vi "长度判断.vi"(6 "输入元素 2":string, 8 "error in (no error)":errorcluster caption="错误输入（无错误）", 9 "压力打印代码据库":string[][](table)=[["C.0A.00D", "C.04.001", "C.0B.31B", ""], ["C.0A.01D", "C.04.002", "C.0B.32B", ""], ["C.0A.02D", "C.04.003", "C.0B.33B", ""], ["C.0A.03D", "C.04.004", "C.0B.34B", ""], ["C.0A.04D", "C.04.005", "C.0B.35B", ""], ["C.0A.05D", "C.04.006", "C.0B.36B", ""], ["C.0A.06D", "C.04.007", "C.0B.37B", ""], ["C.0A.07D", "C.04.008", "C.0B.38B", ""], ["C.0A.08D", "C.04.009", "C.0B.39B", ""], ["C.0A.09D", "C.04.010", "C.0B.3AB", ""], ["C.0A.0AD", "C.04.011", "C.0B.3BB", ""], ["C.0A.0BD", "C.04.012", "C.0B.3CB", ""], ["C.0A.0CD", "C.04.013", "C.0B.1MB", ""], ["C.0A.0DD", "C.04.014", "C.0B.1NB", ""], ["C.0A.0ED", "C.04.015", "C.0B.1PB", ""], ["C.0A.0FD", "C.04.016", "C.0B.1QB", ""], ["C.0A.0GD", "C.04.017", "C.0B.1RB", ""], ["C.0A.0HD", "C.04.018", "C.0B.1SB", ""], ["C.0A.0JD", "C.04.019", "C.0B.1TB", ""], ["C.0A.0KD", "C.04.020", "C.0B.1UB", ""], ["C.0A.0LD", "C.04.021", "C.0B.1VB", ""], ["C.0A.0MD", "C.04.022", "C.0B.1WB", ""], ["C.0A.0ND", "C.04.023", "C.0B.1XB", ""], ["C.0A.0PD", "C.04.024", "C.0B.1YB", ""], ["C.0A.0QD", "C.04.025", "C.0B.1ZB", ""], ["C.0A.0RD", "C.04.026", "C.0B.13B", ""], ["C.0A.0SD", "C.04.027", "C.0B.21B", ""], ["C.0A.0TD", "C.04.028", "C.0B.22B", ""], ["C.0A.0UD", "C.04.029", "C.0B.23B", ""], ["C.0A.0VD", "C.04.030", "C.0B.15B", ""], ["C.0A.0WD", "C.04.031", "C.0B.25B", ""], ["C.0A.0XD", "C.04.032", "C.0B.26B", ""], ["C.0A.0YD", "C.04.033", "C.0B.27B", ""], ["C.0A.0ZD", "C.04.034", "C.0B.17B", ""], ["C.0A.10D", "C.04.035", "C.0B.29B", ""], ["C.0A.11D", "C.04.036", "C.0B.2AB", ""], ["C.0A.12D", "C.04.037", "C.0B.2BB", ""], ["C.0A.13D", "C.04.038", "C.0B.19B", ""], ["C.0A.14D", "C.04.039", "C.0B.2DB", ""], ["C.0A.15D", "C.04.040", "C.0B.2EB", ""], ["C.0A.16D", "C.04.041", "C.0B.2FB", ""], ["C.0A.17D", "C.04.042", "C.0B.2GB", ""], ["C.0A.18D", "C.04.043", "C.0B.1AB", ""], ["C.0A.19D", "C.04.044", "C.0B.1BB", ""], ["C.0A.1AD", "C.04.045", "C.0B.2KB", ""], ["C.0A.1BD", "C.04.046", "C.0B.2LB", ""], ["C.0A.1CD", "C.04.047", "C.0B.2MB", ""], ["C.0A.1DD", "C.04.048", "C.0B.1DB", ""], ["C.0A.1ED", "C.04.049", "C.0B.2PB", ""], ["C.0A.1FD", "C.04.050", "C.0B.2QB", ""], ["C.0A.1GD", "C.04.051", "C.0B.2RB", ""], ["C.0A.1HD", "C.04.052", "C.0B.2SB", ""], ["C.0A.1JD", "C.04.053", "C.0B.2TB", ""], ["C.0A.1KD", "C.04.054", "C.0B.2UB", ""], ["C.0A.1LD", "C.04.055", "C.0B.2VB", ""], ["C.0A.1MD", "C.04.056", "C.0B.2WB", ""], ["C.0A.1ND", "C.04.057", "C.0B.2XB", ""], ["C.0A.1PD", "C.04.058", "C.0B.2YB", ""], ["C.0C.01B", "C.04.059", "C.0B.2ZB", ""], ["C.0C.02B", "C.04.060", "C.0B.30B", ""], ["C.0C.03B", "C.08.001", "C.0B.00N", " "], ["C.0C.04B", "C.08.002", "C.0B.01N", " "], ["C.0C.05B", "C.08.003", "C.0B.02N", " "], ["C.0C.06B", "C.08.004", "C.0B.03N", " "], ["C.0C.07B", "C.08.005", "C.0B.04N", " "], ["C.0C.08B", "C.08.006", "C.0B.05N", " "], ["C.0C.09B", "C.08.007", "C.0B.06N", " "], ["C.0C.10B", "C.08.008", "C.0B.07N", " "], ["C.0C.11B", "C.08.009", "C.0B.08N", " "], ["C.0C.12B", "C.08.010", "C.0B.09N", " "], ["C.0C.13B", "C.08.011", "C.0B.10N", " "], ["C.0C.14B", "C.08.012", "C.0B.11N", " "], ["C.0C.15B", "C.08.013", "C.0B.12N", " "], ["C.0C.16B", "C.08.014", "C.0B.13N", " "], ["C.0C.17B", "C.08.015", "C.0B.14N", " "], ["C.0C.18B", "C.08.016", "C.0B.15N", " "], ["C.0C.19B", "C.08.017", "C.0B.16N", " "], ["C.0C.20B", "C.08.018", "C.0B.17N", " "], ["C.0C.21B", "C.08.019", "C.0B.18N", " "], ["C.0C.22B", "C.08.020", "C.0B.19N", " "], ["C.0C.23B", "C.08.021", "C.0B.20N", " "], ["C.0C.24B", "C.08.022", "C.0B.21N", " "], ["C.0C.25B", "C.08.023", "C.0B.22N", " "], ["C.0C.59B", "C.08.024", "C.0B.23N", " "], ["C.0C.60B", "C.08.025", "C.0B.24N", " "], ["C.0C.61B", "C.08.026", "C.0B.25N", " "], ["C.0C.62B", "C.08.027", "C.0B.26N", " "], ["C.0C.63B", "C.08.028", "C.0B.27N", " "], ["C.0C.64B", "C.08.029", "C.0B.28N", " "], ["C.0C.65B", "C.08.030", "C.0B.29N", " "], ["C.0C.66B", "C.08.031", "C.0B.40E", " "], ["C.0C.67B", "C.08.032", "C.0B.41E", " "], ["C.0C.68B", "C.08.033", "C.0B.02E", " "], ["C.0C.69B", "C.08.034", "C.0B.03E", " "], ["C.0C.70B", "C.08.035", "C.0B.42E", " "], ["C.0C.71B", "C.08.036", "C.0B.43E", " "], ["C.0C.72B", "C.08.037", "C.0B.06E", " "], ["C.0C.73B", "C.08.038", "C.0B.07E", " "], ["C.0C.74B", "C.08.039", "C.0B.44E", " "], ["C.0C.75B", "C.08.040", "C.0B.45E", " "], ["C.0C.76B", "C.08.041", "C.0B.63E", " "], ["C.0C.77B", "C.08.042", "C.0B.11E", " "], ["C.0C.78B", "C.08.043", "C.0B.46E", " "], ["C.0C.01G", "C.08.044", "C.0B.47E", " "], ["C.0C.02G", "C.08.045", "C.0B.64E", " "], ["C.0C.03G", "C.08.046", "C.0B.15E", " "], ["C.0C.04G", "C.08.047", "C.0B.48E", " "], ["C.0C.05G", "C.08.048", "C.0B.49E", " "], ["C.0C.06G", "C.08.049", "C.0B.65E", " "], ["C.0C.07G", "C.08.050", "C.0B.19E", " "], ["C.0C.08G", "C.08.051", "C.0B.50E", " "], ["C.0C.09G", "C.08.052", "C.0B.51E", " "], ["C.0C.10G", "C.08.053", "C.0B.22E", " "], ["C.0C.11G", "C.08.054", "C.0B.23E", " "], ["C.0C.12G", "C.08.055", "C.0B.52E", " "], ["C.0C.13G", "C.08.056", "C.0B.53E", " "], ["C.0C.14G", "C.08.057", "C.0B.26E", " "], ["C.0C.15G", "C.08.058", "C.0B.27E", " "], ["C.0C.16G", "C.08.059", "C.0B.54E", " "], ["C.0C.17G", "C.08.060", "C.0B.30E", " "], ["C.0C.18G", "C.0C.01C", "C.0B.31E", " "], ["C.0C.19G", "C.0C.02C", "C.0B.55E", " "], ["C.0C.20G", "C.0C.03C", "C.0B.56E", " "], ["C.0C.21G", "C.0C.04C", "C.0B.57E", " "], ["C.0C.22G", "C.0C.05C", "C.0B.58E", " "], ["C.0C.23G", "C.0C.06C", "C.0B.34E", " "], ["C.0C.24G", "C.0C.07C", "C.0B.35E", " "], ["C.0C.25G", "C.0C.08C", "C.0B.59E", " "], [" ", "C.0C.09C", "C.0B.60E", " "], [" ", "C.0C.10C", "C.0B.61E", " "], [" ", "C.0C.11C", "C.0B.62E", " "], [" ", "C.0C.12C", "C.0B.38E", " "], [" ", "C.0C.13C", "C.0B.39E", " "], [" ", "C.0C.14C", "C.0B.0QE", " "], [" ", "C.0C.15C", "C.0B.0RE", " "], [" ", "C.0C.16C", "C.0B.0SE", " "], [" ", "C.0C.17C", "C.0B.0TE", " "], [" ", "C.0C.18C", "C.0B.0UE", " "], [" ", "C.0C.19C", "C.0B.0VE", " "], [" ", "C.0C.20C", "C.0B.0WE", " "], [" ", "C.0C.21C", "C.0B.0XE", " "], [" ", "C.0C.22C", "C.0B.0YE", " "], [" ", "C.0C.23C", "C.0B.0ZE", " "], [" ", "C.0C.24C", "C.0B.10E", " "], [" ", "C.0C.25C", "C.0B.11E", " "], [" ", "C.0C.26C", "C.0B.12E", " "], [" ", "C.0C.27C", "C.0B.13E", " "], [" ", "C.0C.28C", "C.0B.14E", " "], [" ", "C.0C.29C", "C.0B.15E", " "], [" ", "C.0C.30C", "C.0B.16E", " "], [" ", "C.0C.31C", "C.0B.17E", " "], [" ", "C.0C.32C", "C.0B.18E", " "], [" ", "C.0C.33C", "C.0B.19E", " "], [" ", "C.0C.34C", "C.0B.1AE", " "], [" ", "C.0C.35C", "C.0B.1BE", " "], [" ", "C.0C.36C", "C.0B.1CE", " "], [" ", "C.0C.37C", "C.0B.1DE", " "], [" ", "C.0C.38C", "C.0B.1EE", " "], [" ", "C.0C.39C", "C.0B.1FE", " "], [" ", "C.0C.40C", "C.0B.1GE", " "], [" ", "C.0C.41C", "C.0B.1HE", " "], [" ", "C.0C.42C", "C.0B.1KE", " "], [" ", "C.0C.43C", "C.0B.1LE", " "], [" ", "C.0C.44C", "C.0B.1NE", " "], [" ", "C.0C.45C", "C.0B.1QE", " "], [" ", "C.0C.46C", "C.0B.1SE", " "], [" ", "C.0C.47C", " ", ""], [" ", "C.0C.48C", " ", ""], [" ", "C.0C.49C", " ", ""], [" ", "C.0C.50C", " ", ""], [" ", "C.0C.51C", " ", ""], [" ", "C.0C.52C", " ", ""], [" ", "C.0C.53C", " ", ""], [" ", "C.0C.54C", " ", ""], [" ", "C.0C.55C", " ", ""], [" ", "C.0C.56C", " ", ""], [" ", "C.0C.57C", " ", ""], [" ", "C.0C.58C", " ", ""], [" ", "C.0C.59C", " ", ""], [" ", "C.0C.60C", " ", ""], [" ", "C.0C.01E", " ", ""], [" ", "C.0C.02E", " ", ""], [" ", "C.0C.03E", " ", ""], [" ", "C.0C.04E", " ", ""], [" ", "C.0C.05E", " ", ""], [" ", "C.0C.06E", " ", ""], [" ", "C.0C.07E", " ", ""], [" ", "C.0C.08E", " ", ""], [" ", "C.0C.09E", " ", ""], [" ", "C.0C.10E", " ", ""], [" ", "C.0C.11E", " ", ""], [" ", "C.0C.12E", " ", ""], [" ", "C.0C.13E", " ", ""], [" ", "C.0C.14E", " ", ""], [" ", "C.0C.15E", " ", ""], [" ", "C.0C.16E", " ", ""], [" ", "C.0C.17E", " ", ""], [" ", "C.0C.18E", " ", ""], [" ", "C.0C.19E", " ", ""], [" ", "C.0C.20E", " ", ""], [" ", "C.0C.21E", " ", ""], [" ", "C.0C.22E", " ", ""], [" ", "C.0C.23E", " ", ""], [" ", "C.0C.24E", " ", ""], [" ", "C.0C.25E", " ", ""], [" ", "C.0C.26E", " ", ""], [" ", "C.0C.27E", " ", ""], [" ", "C.0C.28E", " ", ""], [" ", "C.0C.29E", " ", ""], [" ", "C.0C.30E", " ", ""], [" ", "C.0C.31E", " ", ""], [" ", "C.0C.32E", " ", ""], [" ", "C.0C.33E", " ", ""], [" ", "C.0C.34E", " ", ""], [" ", "C.0C.35E", " ", ""], [" ", "C.0C.36E", " ", ""], [" ", "C.0C.37E", " ", ""], [" ", "C.0C.38E", " ", ""], [" ", "C.0C.39E", " ", ""], [" ", "C.0C.40E", " ", ""], [" ", "C.0C.41E", " ", ""], [" ", "C.0C.42E", " ", ""], [" ", "C.0C.43E", " ", ""], [" ", "C.0C.44E", " ", ""], [" ", "C.0C.45E", " ", ""], [" ", "C.0C.46E", " ", ""], [" ", "C.0C.47E", " ", ""], [" ", "C.0C.48E", " ", ""], [" ", "C.0C.49E", " ", ""], [" ", "C.0C.50E", " ", ""], [" ", "C.0C.51E", " ", ""], [" ", "C.0C.52E", " ", ""], [" ", "C.0C.53E", " ", ""], [" ", "C.0C.54E", " ", ""], [" ", "C.0C.55E", " ", ""], [" ", "C.0C.56E", " ", ""], [" ", "C.0C.57E", " ", ""], [" ", "C.0C.58E", " ", ""], [" ", "C.0C.59E", " ", ""], [" ", "C.0C.60E", " ", ""]], 10 "压力表数据库":string[][](table)=[["C.0C.01B", "C.0C.19B", "C.0C.01C", "C.0C.19C", "C.0B.0QE", "C.0B.40E"], ["C.0C.02B", "C.0C.74B", "C.0C.02C", "C.0C.20C", "C.0B.0RE", "C.0B.41E"], ["C.0C.03B", "C.0C.24B", "C.0C.03C", "C.0C.21C", "C.0B.0SE", "C.0B.02E"], ["C.0C.04B", "C.0C.20B", "C.0C.04C", "C.0C.22C", "C.0B.0TE", "C.0B.03E"], ["C.0C.05B", "C.0C.78B", "C.0C.05C", "C.0C.23C", "C.0B.0UE", "C.0B.42E"], ["C.0C.06B", "C.0C.25B", "C.0C.06C", "C.0C.24C", "C.0B.0VE", "C.0B.43E"], ["C.0C.07B", "C.0C.19G", "C.0C.07C", "C.0C.25C", "C.0B.0WE", "C.0B.06E"], ["C.0C.08B", "C.0C.20G", "C.0C.08C", "C.0C.26C", "C.0B.0XE", "C.0B.07E"], ["C.0C.09B", "C.0C.24G", "C.0C.09C", "C.0C.27C", "C.0B.0YE", "C.0B.44E"], ["C.0C.10B", "C.0C.25G", "C.0C.10C", "C.0C.28C", "C.0B.0ZE", "C.0B.45E"], ["C.0C.11B", "C.0A.0JD", "C.0C.11C", "C.0C.30C", "C.0B.10E", "C.0B.63E"], ["C.0C.12B", "C.0A.0KD", "C.0C.12C", "C.0C.51C", "C.0B.11E", "C.0B.11E"], ["C.0C.13B", "C.0A.0PD", "C.0C.13C", "C.0C.52C", "C.0B.12E", "C.0B.46E"], ["C.0C.14B", "C.0A.0QD", "C.0C.14C", "C.0C.53C", "C.0B.13E", "C.0B.47E"], ["C.0C.15B", "C.0A.16D", "C.0C.15C", "C.0C.54C", "C.0B.14E", "C.0B.64E"], ["C.0C.16B", "C.0A.1AD", "C.0C.16C", "C.0C.55C", "C.0B.15E", "C.0B.15E"], ["C.0C.17B", "", "C.0C.17C", "C.0C.56C", "C.0B.16E", "C.0B.04F"], ["C.0C.18B", "", "C.0C.18C", "C.0C.57C", "C.0B.17E", "C.0B.05F"], ["C.0C.21B", "", "C.0C.31C", "C.0C.58C", "C.0B.18E", "C.0B.06F"], ["C.0C.22B", "", "C.0C.32C", "C.0C.59C", "C.0B.19E", "C.0B.07F"], ["C.0C.23B", "", "C.0C.33C", "C.0C.60C", "C.0B.1AE", "C.0B.08F"], ["C.0C.59B", "", "C.0C.34C", "C.0C.19E", "C.0B.1BE", "C.0B.09F"], ["C.0C.60B", "", "C.0C.35C", "C.0C.20E", "C.0B.1CE", "C.0B.10F"], ["C.0C.61B", "", "C.0C.36C", "C.0C.21E", "C.0B.1DE", "C.0B.11F"], ["C.0C.62B", "", "C.0C.37C", "C.0C.22E", "C.0B.1EE", "C.0B.12F"], ["C.0C.63B", "", "C.0C.38C", "C.0C.23E", "C.0B.1FE", "C.0B.13F"], ["C.0C.64B", "", "C.0C.39C", "C.0C.24E", "C.0B.1GE", "C.0B.14F"], ["C.0C.65B", "", "C.0C.40C", "C.0C.25E", "C.0B.1HE", "C.0B.15F"], ["C.0C.66B", "", "C.0C.41C", "C.0C.26E", "C.0B.1KE", ""], ["C.0C.67B", "", "C.0C.42C", "C.0C.27E", "C.0B.1LE", ""], ["C.0C.68B", "", "C.0C.43C", "C.0C.28E", "C.0B.1NE", ""], ["C.0C.69B", "", "C.0C.44C", "C.0C.51E", "C.0B.1QE", ""], ["C.0C.70B", "", "C.0C.45C", "C.0C.52E", "C.0B.1SE", ""], ["C.0C.71B", "", "C.0C.46C", "C.0C.53E", "C.0B.1EE", ""], ["C.0C.72B", "", "C.0C.47C", "C.0C.54E", "C.0B.1FE", ""], ["C.0C.73B", "", "C.0C.48C", "C.0C.55E", "C.0B.0QE", ""], ["C.0C.75B", "", "C.0C.49C", "C.0C.56E", "C.0B.0RE", ""], ["C.0C.76B", "", "C.0C.50C", "C.0C.57E", "C.0B.1GE", ""], ["C.0C.77B", "", "C.0C.29C", "C.0C.58E", "C.0B.1HE", ""], ["C.0C.01G", "", "C.0C.01E", "C.0C.59E", "C.0B.0UE", ""], ["C.0C.02G", "", "C.0C.02E", "C.0C.60E", "C.0B.0VE", ""], ["C.0C.03G", "", "C.0C.03E", "C.0C.19H", "C.0B.0WE", ""], ["C.0C.04G", "", "C.0C.04E", "C.0C.20H", "C.0B.1KE", ""], ["C.0C.05G", "", "C.0C.05E", "C.0C.21H", "C.0B.1LE", ""], ["C.0C.06G", "", "C.0C.06E", "C.0C.22H", "C.0B.0YE", ""], ["C.0C.07G", "", "C.0C.07E", "C.0C.23H", "C.0B.0ZE", ""], ["C.0C.08G", "", "C.0C.08E", "C.0C.24H", "C.0B.10E", ""], ["C.0C.09G", "", "C.0C.09E", "C.0C.25H", "C.0B.1NE", ""], ["C.0C.10G", "", "C.0C.10E", "C.0C.26H", "C.0B.12E", ""], ["C.0C.11G", "", "C.0C.11E", "C.0C.27H", "C.0B.13E", ""], ["C.0C.12G", "", "C.0C.12E", "C.0C.28H", "C.0B.14E", ""], ["C.0C.13G", "", "C.0C.13E", "C.0C.29H", "C.0B.1QE", ""], ["C.0C.14G", "", "C.0C.14E", "C.0C.30H", "C.0B.16E", ""], ["C.0C.15G", "", "C.0C.15E", "", "C.0B.17E", ""], ["C.0C.16G", "", "C.0C.16E", "", "C.0B.18E", ""], ["C.0C.17G", "", "C.0C.17E", "", "C.0B.1SE", ""], ["C.0C.18G", "", "C.0C.18E", "", "C.0B.1AE", ""], ["C.0C.21G", "", "C.0C.29E", "", "C.0B.1BE", ""], ["C.0C.22G", "", "C.0C.30E", "", "C.0B.1CE", ""], ["C.0C.23G", "", "C.0C.31E", "", "C.0B.31B", ""], ["C.0A.00D", "", "C.0C.32E", "", "C.0B.32B", ""], ["C.0A.01D", "", "C.0C.33E", "", "C.0B.33B", ""], ["C.0A.02D", "", "C.0C.34E", "", "C.0B.34B", ""], ["C.0A.03D", "", "C.0C.35E", "", "C.0B.35B", ""], ["C.0A.04D", "", "C.0C.36E", "", "C.0B.36B", ""], ["C.0A.05D", "", "C.0C.37E", "", "C.0B.37B", ""], ["C.0A.06D", "", "C.0C.38E", "", "C.0B.38B", ""], ["C.0A.07D", "", "C.0C.39E", "", "C.0B.39B", ""], ["C.0A.08D", "", "C.0C.40E", "", "C.0B.3AB", ""], ["C.0A.09D", "", "C.0C.41E", "", "C.0B.3BB", ""], ["C.0A.0AD", "", "C.0C.42E", "", "C.0B.3CB", ""], ["C.0A.0BD", "", "C.0C.43E", "", "C.0B.1EB", ""], ["C.0A.0CD", "", "C.0C.44E", "", "C.0B.1FB", ""], ["C.0A.0DD", "", "C.0C.45E", "", "C.0B.1GB", ""], ["C.0A.0ED", "", "C.0C.46E", "", "C.0B.12B", ""], ["C.0A.0FD", "", "C.0C.47E", "", "C.0B.1HB", ""], ["C.0A.0GD", "", "C.0C.48E", "", "C.0B.14B", ""], ["C.0A.0HD", "", "C.0C.49E", "", "C.0B.1JB", ""], ["C.0A.0LD", "", "C.0C.50E", "", "C.0B.16B", ""], ["C.0A.0MD", "", "C.0C.51E", "", "C.0B.1KB", ""], ["C.0A.0ND", "", "C.0C.52E", "", "C.0B.18B", ""], ["C.0A.0RD", "", "C.0C.53E", "", "C.0B.1LB", ""], ["C.0A.0SD", "", "C.0C.54E", "", "C.0B.1CB", ""], ["C.0A.0TD", "", "C.0C.55E", "", "C.0B.1MB", ""], ["C.0A.0UD", "", "C.0C.56E", "", "C.0B.1NB", ""], ["C.0A.0VD", "", "C.0C.57E", "", "C.0B.1PB", ""], ["C.0A.0WD", "", "C.0C.58E", "", "C.0B.1QB", ""], ["C.0A.0XD", "", "C.0C.59E", "", "C.0B.1RB", ""], ["C.0A.0YD", "", "C.0C.60E", "", "C.0B.1SB", ""], ["C.0A.0ZD", "", "C.0C.01H", "", "C.0B.1TB", ""], ["C.0A.10D", "", "C.0C.02H", "", "C.0B.1UB", ""], ["C.0A.11D", "", "C.0C.03H", "", "C.0B.1VB", ""], ["C.0A.12D", "", "C.0C.04H", "", "C.0B.1WB", ""], ["C.0A.13D", "", "C.0C.05H", "", "C.0B.1XB", ""], ["C.0A.14D", "", "C.0C.06H", "", "C.0B.1YB", ""], ["C.0A.15D", "", "C.0C.07H", "", "C.0B.1ZB", ""], ["C.0A.17D", "", "C.0C.08H", "", "C.0B.13B", ""], ["C.0A.18D", "", "C.0C.09H", "", "C.0B.21B", ""], ["C.0A.19D", "", "C.0C.10H", "", "C.0B.22B", ""], ["C.0A.1BD", "", "C.0C.11H", "", "C.0B.23B", ""], ["C.0A.1CD", "", "C.0C.12H", "", "C.0B.15B", ""], ["C.0A.1DD", "", "C.0C.13H", "", "C.0B.25B", ""], ["C.0A.1ED", "", "C.0C.14H", "", "C.0B.26B", ""], ["C.0A.1FD", "", "C.0C.15H", "", "C.0B.27B", ""], ["C.0A.1GD", "", "C.0C.16H", "", "C.0B.17B", ""], ["C.0A.1HD", "", "C.0C.17H", "", "C.0B.29B", ""], ["C.0A.1JD", "", "C.0C.18H", "", "C.0B.2AB", ""], ["C.0A.1KD", "", "C.0C.19H", "", "C.0B.2BB", ""], ["C.0A.1LD", "", "C.0C.20H", "", "C.0B.19B", ""], ["C.0A.1MD", "", "C.0C.21H", "", "C.0B.2DB", ""], ["C.0A.1ND", "", "C.0C.22H", "", "C.0B.2EB", ""], ["C.0A.1PD", "", "C.0C.23H", "", "C.0B.2FB", ""], ["", "", "C.0C.24H", "", "C.0B.2GB", ""], ["", "", "C.0C.25H", "", "C.0B.1AB", ""], ["", "", "C.0C.26H", "", "C.0B.1BB", ""], ["", "", "C.0C.27H", "", "C.0B.2KB", ""], ["", "", "C.0C.28H", "", "C.0B.2LB", ""], ["", "", "C.0C.29H", "", "C.0B.2MB", ""], ["", "", "C.0C.30H", "", "C.0B.1DB", ""], ["", "", "C.04.001", "", "C.0B.2PB", ""], ["", "", "C.04.002", "", "C.0B.2QB", ""], ["", "", "C.04.003", "", "C.0B.2RB", ""], ["", "", "C.04.004", "", "C.0B.2SB", ""], ["", "", "C.04.005", "", "C.0B.2TB", ""], ["", "", "C.04.006", "", "C.0B.2UB", ""], ["", "", "C.04.007", "", "C.0B.2VB", ""], ["", "", "C.04.008", "", "C.0B.2WB", ""], ["", "", "C.04.009", "", "C.0B.2XB", ""], ["", "", "C.04.010", "", "C.0B.2YB", ""], ["", "", "C.04.011", "", "C.0B.2ZB", ""], ["", "", "C.04.012", "", "C.0B.30B", ""], ["", "", "C.04.013", "", "C.0B.48E", ""], ["", "", "C.04.014", "", "C.0B.49E", ""], ["", "", "C.04.015", "", "C.0B.65E", ""], ["", "", "C.04.016", "", "C.0B.19E", ""], ["", "", "C.04.017", "", "C.0B.50E", ""], ["", "", "C.04.018", "", "C.0B.51E", ""], ["", "", "C.04.019", "", "C.0B.22E", ""], ["", "", "C.04.020", "", "C.0B.23E", ""], ["", "", "C.04.021", "", "C.0B.52E", ""], ["", "", "C.04.022", "", "C.0B.53E", ""], ["", "", "C.04.023", "", "C.0B.26E", ""], ["", "", "C.04.024", "", "C.0B.27E", ""], ["", "", "C.04.025", "", "C.0B.54E", ""], ["", "", "C.04.026", "", "C.0B.30E", ""], ["", "", "C.04.027", "", "C.0B.31E", ""], ["", "", "C.04.028", "", "C.0B.55E", ""], ["", "", "C.04.029", "", "C.0B.56E", ""], ["", "", "C.04.030", "", "C.0B.57E", ""], ["", "", "C.04.031", "", "C.0B.58E", ""], ["", "", "C.04.032", "", "C.0B.34E", ""], ["", "", "C.04.033", "", "C.0B.35E", ""], ["", "", "C.04.034", "", "C.0B.59E", ""], ["", "", "C.04.035", "", "C.0B.60E", ""], ["", "", "C.04.036", "", "C.0B.61E", ""], ["", "", "C.04.037", "", "C.0B.62E", ""], ["", "", "C.04.038", "", "C.0B.38E", ""], ["", "", "C.04.039", "", "C.0B.39E", ""], ["", "", "C.04.040", "", "C.0B.16F", ""], ["", "", "C.04.041", "", "C.0B.17F", ""], ["", "", "C.04.042", "", "C.0B.18F", ""], ["", "", "C.04.043", "", "C.0B.19F", ""], ["", "", "C.04.044", "", "C.0B.20F", ""], ["", "", "C.04.045", "", "C.0B.21F", ""], ["", "", "C.04.046", "", "C.0B.22F", ""], ["", "", "C.04.047", "", "C.0B.23F", ""], ["", "", "C.04.048", "", "C.0B.24F", ""], ["", "", "C.04.049", "", "C.0B.25F", ""], ["", "", "C.04.050", "", "C.0B.26F", ""], ["", "", "C.04.051", "", "C.0B.27F", ""], ["", "", "C.04.052", "", "C.0B.28F", ""], ["", "", "C.04.053", "", "C.0B.29F", ""], ["", "", "C.04.054", "", "C.0B.30F", ""], ["", "", "C.04.055", "", "C.0B.31F", ""], ["", "", "C.04.056", "", "C.0B.32F", ""], ["", "", "C.04.057", "", "C.0B.33F", ""], ["", "", "C.04.058", "", "C.0B.34F", ""], ["", "", "C.04.059", "", "C.0B.35F", ""], ["", "", "C.04.060", "", "C.0B.36F", ""], ["", "", "C.08.001", "", "C.0B.37F", ""], ["", "", "C.08.002", "", "C.0B.38F", ""], ["", "", "C.08.003", "", "C.0B.39F", ""], ["", "", "C.08.004", "", "C.0B.40F", ""], ["", "", "C.08.005", "", "C.0B.41F", ""], ["", "", "C.08.006", "", "C.0B.42F", ""], ["", "", "C.08.007", "", "C.0B.30B", ""], ["", "", "C.08.008", "", "C.0B.2ZB", ""], ["", "", "C.08.009", "", "C.0B.2YB", ""], ["", "", "C.08.010", "", "C.0B.2XB", ""], ["", "", "C.08.011", "", "C.0B.2WB", ""], ["", "", "C.08.012", "", "C.0B.2VB", ""], ["", "", "C.08.013", "", "C.0B.2UB", ""], ["", "", "C.08.014", "", "C.0B.2TB", ""], ["", "", "C.08.015", "", "C.0B.2SB", ""], ["", "", "C.08.016", "", "C.0B.2RB", ""], ["", "", "C.08.017", "", "C.0B.2QB", ""], ["", "", "C.08.018", "", "C.0B.2PB", ""], ["", "", "C.08.019", "", "C.0B.1DB", ""], ["", "", "C.08.020", "", "C.0B.1CB", ""], ["", "", "C.08.021", "", "C.0B.2MB", ""], ["", "", "C.08.022", "", "C.0B.1LB", ""], ["", "", "C.08.023", "", "C.0B.2LB", ""], ["", "", "C.08.024", "", "C.0B.2KB", ""], ["", "", "C.08.025", "", "C.0B.1BB", ""], ["", "", "C.08.026", "", "C.0B.1AB", ""], ["", "", "C.08.027", "", "C.0B.2GB", ""], ["", "", "C.08.028", "", "C.0B.2FB", ""], ["", "", "C.08.029", "", "C.0B.2EB", ""], ["", "", "C.08.030", "", "C.0B.2DB", ""], ["", "", "C.08.031", "", "C.0B.19B", ""], ["", "", "C.08.032", "", "C.0B.18B", ""], ["", "", "C.08.033", "", "C.0B.2BB", ""], ["", "", "C.08.034", "", "C.0B.1KB", ""], ["", "", "C.08.035", "", "C.0B.2AB", ""], ["", "", "C.08.036", "", "C.0B.29B", ""], ["", "", "C.08.037", "", "C.0B.17B", ""], ["", "", "C.08.038", "", "C.0B.16B", ""], ["", "", "C.08.039", "", "C.0B.27B", ""], ["", "", "C.08.040", "", "C.0B.1JB", ""], ["", "", "C.08.041", "", "C.0B.26B", ""], ["", "", "C.08.042", "", "C.0B.25B", ""], ["", "", "C.08.043", "", "C.0B.15B", ""], ["", "", "C.08.044", "", "C.0B.14B", ""], ["", "", "C.08.045", "", "C.0B.23B", ""], ["", "", "C.08.046", "", "C.0B.1HB", ""], ["", "", "C.08.047", "", "C.0B.22B", ""], ["", "", "C.08.048", "", "C.0B.21B", ""], ["", "", "C.08.049", "", "C.0B.13B", ""], ["", "", "C.08.050", "", "C.0B.12B", ""], ["", "", "C.08.051", "", "C.0B.1ZB", ""], ["", "", "C.08.052", "", "C.0B.1GB", ""], ["", "", "C.08.053", "", "C.0B.1YB", ""], ["", "", "C.08.054", "", "C.0B.1XB", ""], ["", "", "C.08.055", "", "C.0B.1WB", ""], ["", "", "C.08.056", "", "C.0B.1FB", ""], ["", "", "C.08.057", "", "C.0B.1VB", ""], ["", "", "C.08.058", "", "C.0B.1EB", ""], ["", "", "C.08.059", "", "C.0B.1UB", ""], ["", "", "C.08.060", "", "C.0B.1TB", ""], ["", "", "", "", "C.0B.1SB", ""], ["", "", "", "", "C.0B.1RB", ""], ["", "", "", "", "C.0B.1QB", ""], ["", "", "", "", "C.0B.1PB", ""], ["", "", "", "", "C.0B.1NB", ""], ["", "", "", "", "C.0B.1MB", ""], ["", "", "", "", "C.0B.3CB", ""], ["", "", "", "", "C.0B.3BB", ""], ["", "", "", "", "C.0B.3AB", ""], ["", "", "", "", "C.0B.39B", ""], ["", "", "", "", "C.0B.38B", ""], ["", "", "", "", "C.0B.37B", ""], ["", "", "", "", "C.0B.36B", ""], ["", "", "", "", "C.0B.35B", ""], ["", "", "", "", "C.0B.34B", ""], ["", "", "", "", "C.0B.33B", ""], ["", "", "", "", "C.0B.32B", ""], ["", "", "", "", "C.0B.31B", ""], ["", "", "", "", "C.0B.1TE", ""], ["", "", "", "", "C.0B.1DE", ""], ["", "", "", "", "C.0B.1CE", ""], ["", "", "", "", "C.0B.1BE", ""], ["", "", "", "", "C.0B.1AE", ""], ["", "", "", "", "C.0B.1SE", ""], ["", "", "", "", "C.0B.18E", ""], ["", "", "", "", "C.0B.17E", ""], ["", "", "", "", "C.0B.16E", ""], ["", "", "", "", "C.0B.1QE", ""], ["", "", "", "", "C.0B.14E", ""], ["", "", "", "", "C.0B.13E", ""], ["", "", "", "", "C.0B.12E", ""], ["", "", "", "", "C.0B.1NE", ""], ["", "", "", "", "C.0B.10E", ""], ["", "", "", "", "C.0B.0ZE", ""], ["", "", "", "", "C.0B.0YE", ""], ["", "", "", "", "C.0B.1LE", ""], ["", "", "", "", "C.0B.1KE", ""], ["", "", "", "", "C.0B.0WE", ""], ["", "", "", "", "C.0B.0VE", ""], ["", "", "", "", "C.0B.0UE", ""], ["", "", "", "", "C.0B.1HE", ""], ["", "", "", "", "C.0B.1GE", ""], ["", "", "", "", "C.0B.0RE", ""], ["", "", "", "", "C.0B.0QE", ""], ["", "", "", "", "C.0B.1FE", ""], ["", "", "", "", "C.0B.1EE", ""]], 11 "输入元素":string) -> (0 "error out":errorcluster caption="错误输出", 1 "压力表打印代码":string, 2 "产品种类":string, 3 "压力表有无判定":string)   [LabVIEW 2017]
panel:
  out "P-B6":string[](array[string])
  out "P-B5":string[](array[string])
  out "P-B4":string[](array[string])
  out "P-B3":string[](array[string])
  out "P-B2":string[](array[string])
  out "P-B1":string[](array[string])
  out "P-A6":string[](array[string])
  out "P-A5":string[](array[string])
  out "P-A4":string[](array[string])
  out "P-A3":string[](array[string])
  out "P-A2":string[](array[string])
  out "P-A1":string[](array[string])
  in  "压力表打印代码据库":string[][](table)=[["C.0C.01E", "C.0C.04E", "C.0C.09E", "C.0C.14E", "C.0C.19E", "C.0C.24E", "C.08.001", "C.08.008", "C.08.017", "C.08.028", "C.08.039", "C.08.050"], ["C.0C.02E", "C.0C.05E", "C.0C.10E", "C.0C.15E", "C.0C.20E", "C.0C.25E", "C.08.002", "C.08.009", "C.08.018", "C.08.029", "C.08.040", "C.08.051"], ["C.0C.03E", "C.0C.06E", "C.0C.11E", "C.0C.16E", "C.0C.21E", "C.0C.26E", "C.08.003", "C.08.010", "C.08.019", "C.08.030", "C.08.041", "C.08.052"], ["C.0C.34E", "C.0C.07E", "C.0C.12E", "C.0C.17E", "C.0C.22E", "C.0C.27E", "C.08.004", "C.08.011", "C.08.020", "C.08.031", "C.08.042", "C.08.053"], ["C.0C.35E", "C.0C.08E", "C.0C.13E", "C.0C.18E", "C.0C.23E", "C.0C.28E", "C.08.005", "C.08.012", "C.08.021", "C.08.032", "C.08.043", "C.08.054"], ["C.0C.36E", "C.0C.31E", "C.0C.32E", "C.0C.29E", "C.0C.30E", "C.0C.33E", "C.08.006", "C.08.013", "C.08.022", "C.08.033", "C.08.044", "C.08.055"], ["C.0C.01H", "C.0C.37E", "C.0C.41E", "C.0C.46E", "C.0C.51E", "C.0C.56E", "C.08.007", "C.08.014", "C.08.023", "C.08.034", "C.08.045", "C.08.056"], ["C.0C.02H", "C.0C.38E", "C.0C.42E", "C.0C.47E", "C.0C.52E", "C.0C.57E", "", "C.08.015", "C.08.024", "C.08.035", "C.08.046", "C.08.057"], ["C.0C.03H", "C.0C.39E", "C.0C.43E", "C.0C.48E", "C.0C.53E", "C.0C.58E", "", "C.08.016", "C.08.025", "C.08.036", "C.08.047", "C.08.058"], ["", "C.0C.40E", "C.0C.44E", "C.0C.49E", "C.0C.54E", "C.0C.59E", "", "", "C.08.026", "C.08.037", "C.08.048", "C.08.059"], ["", "C.0C.04H", "C.0C.45E", "C.0C.50E", "C.0C.55E", "C.0C.60E", "", "", "C.08.027", "C.08.038", "C.08.049", "C.08.060"], ["", "C.0C.05H", "C.0C.09H", "C.0C.14H", "C.0C.19H", "C.0C.24H", "", "", "", "", "", ""], ["", "C.0C.06H", "C.0C.10H", "C.0C.15H", "C.0C.20H", "C.0C.25H", "", "", "", "", "", ""], ["", "C.0C.07H", "C.0C.11H", "C.0C.16H", "C.0C.21H", "C.0C.26H", "", "", "", "", "", ""], ["", "C.0C.08H", "C.0C.12H", "C.0C.17H", "C.0C.22H", "C.0C.27H", "", "", "", "", "", ""], ["", "", "C.0C.13H", "C.0C.18H", "C.0C.23H", "C.0C.28H", "", "", "", "", "", ""], ["", "", "", "C.0C.29H", "C.0C.30H", "", "", "", "", "", "", ""]]
  out "C2":string[](array[string])
  out "C1":string[](array[string])
  out "B2":string[](array[string])
  out "B1":string[](array[string])
  out "A2":string[](array[string])
  out "A1":string[](array[string])
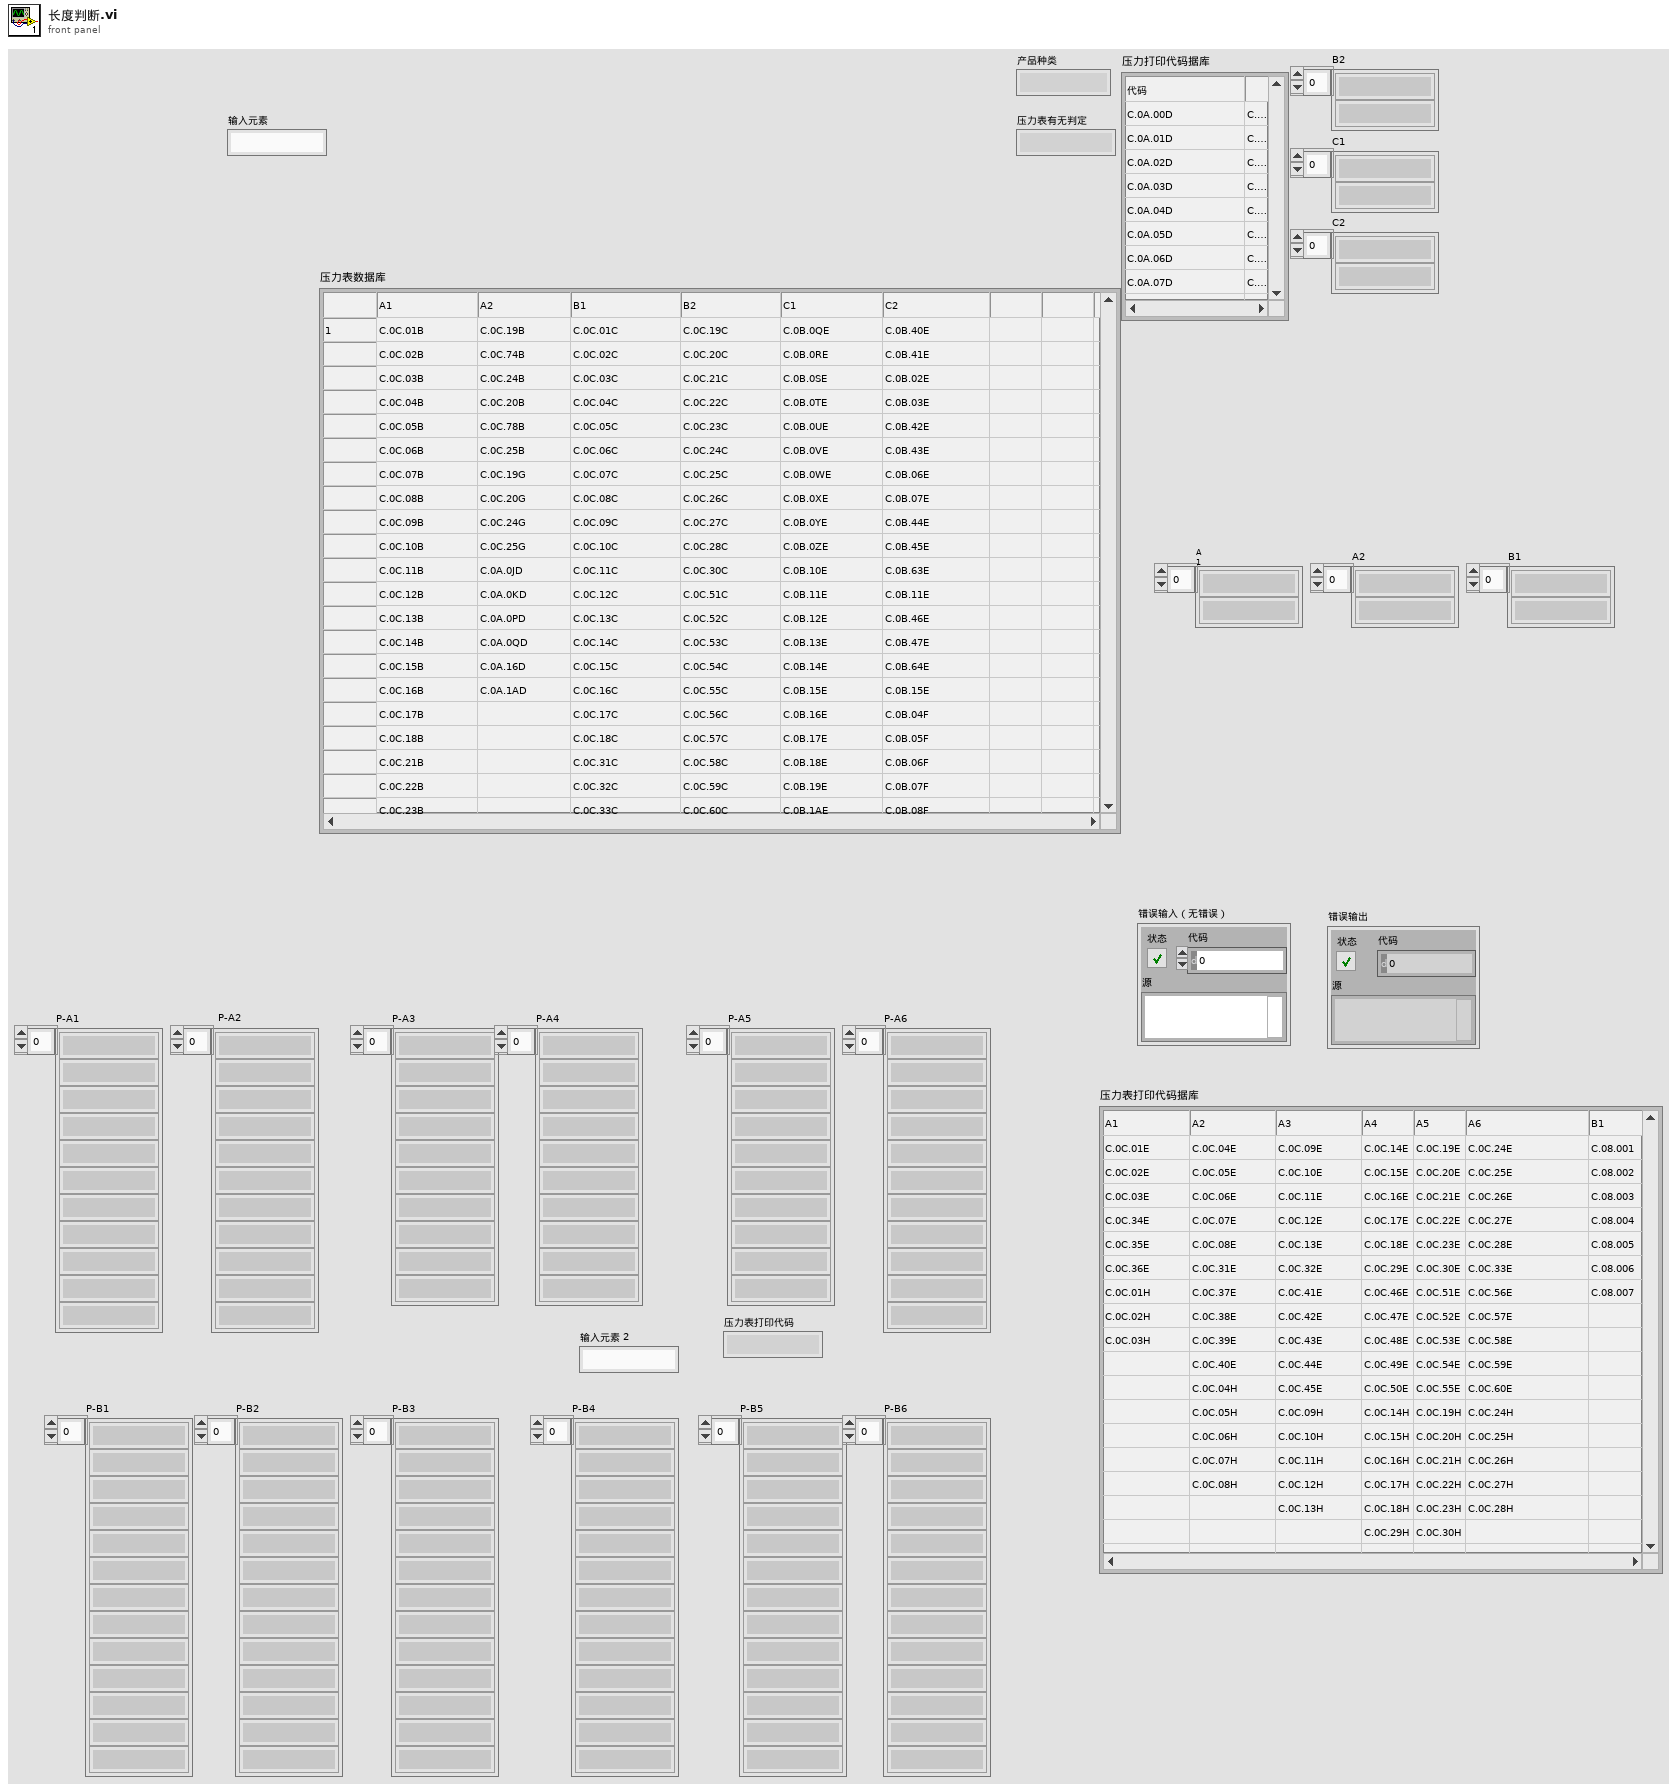
[diagram p1: front panel]
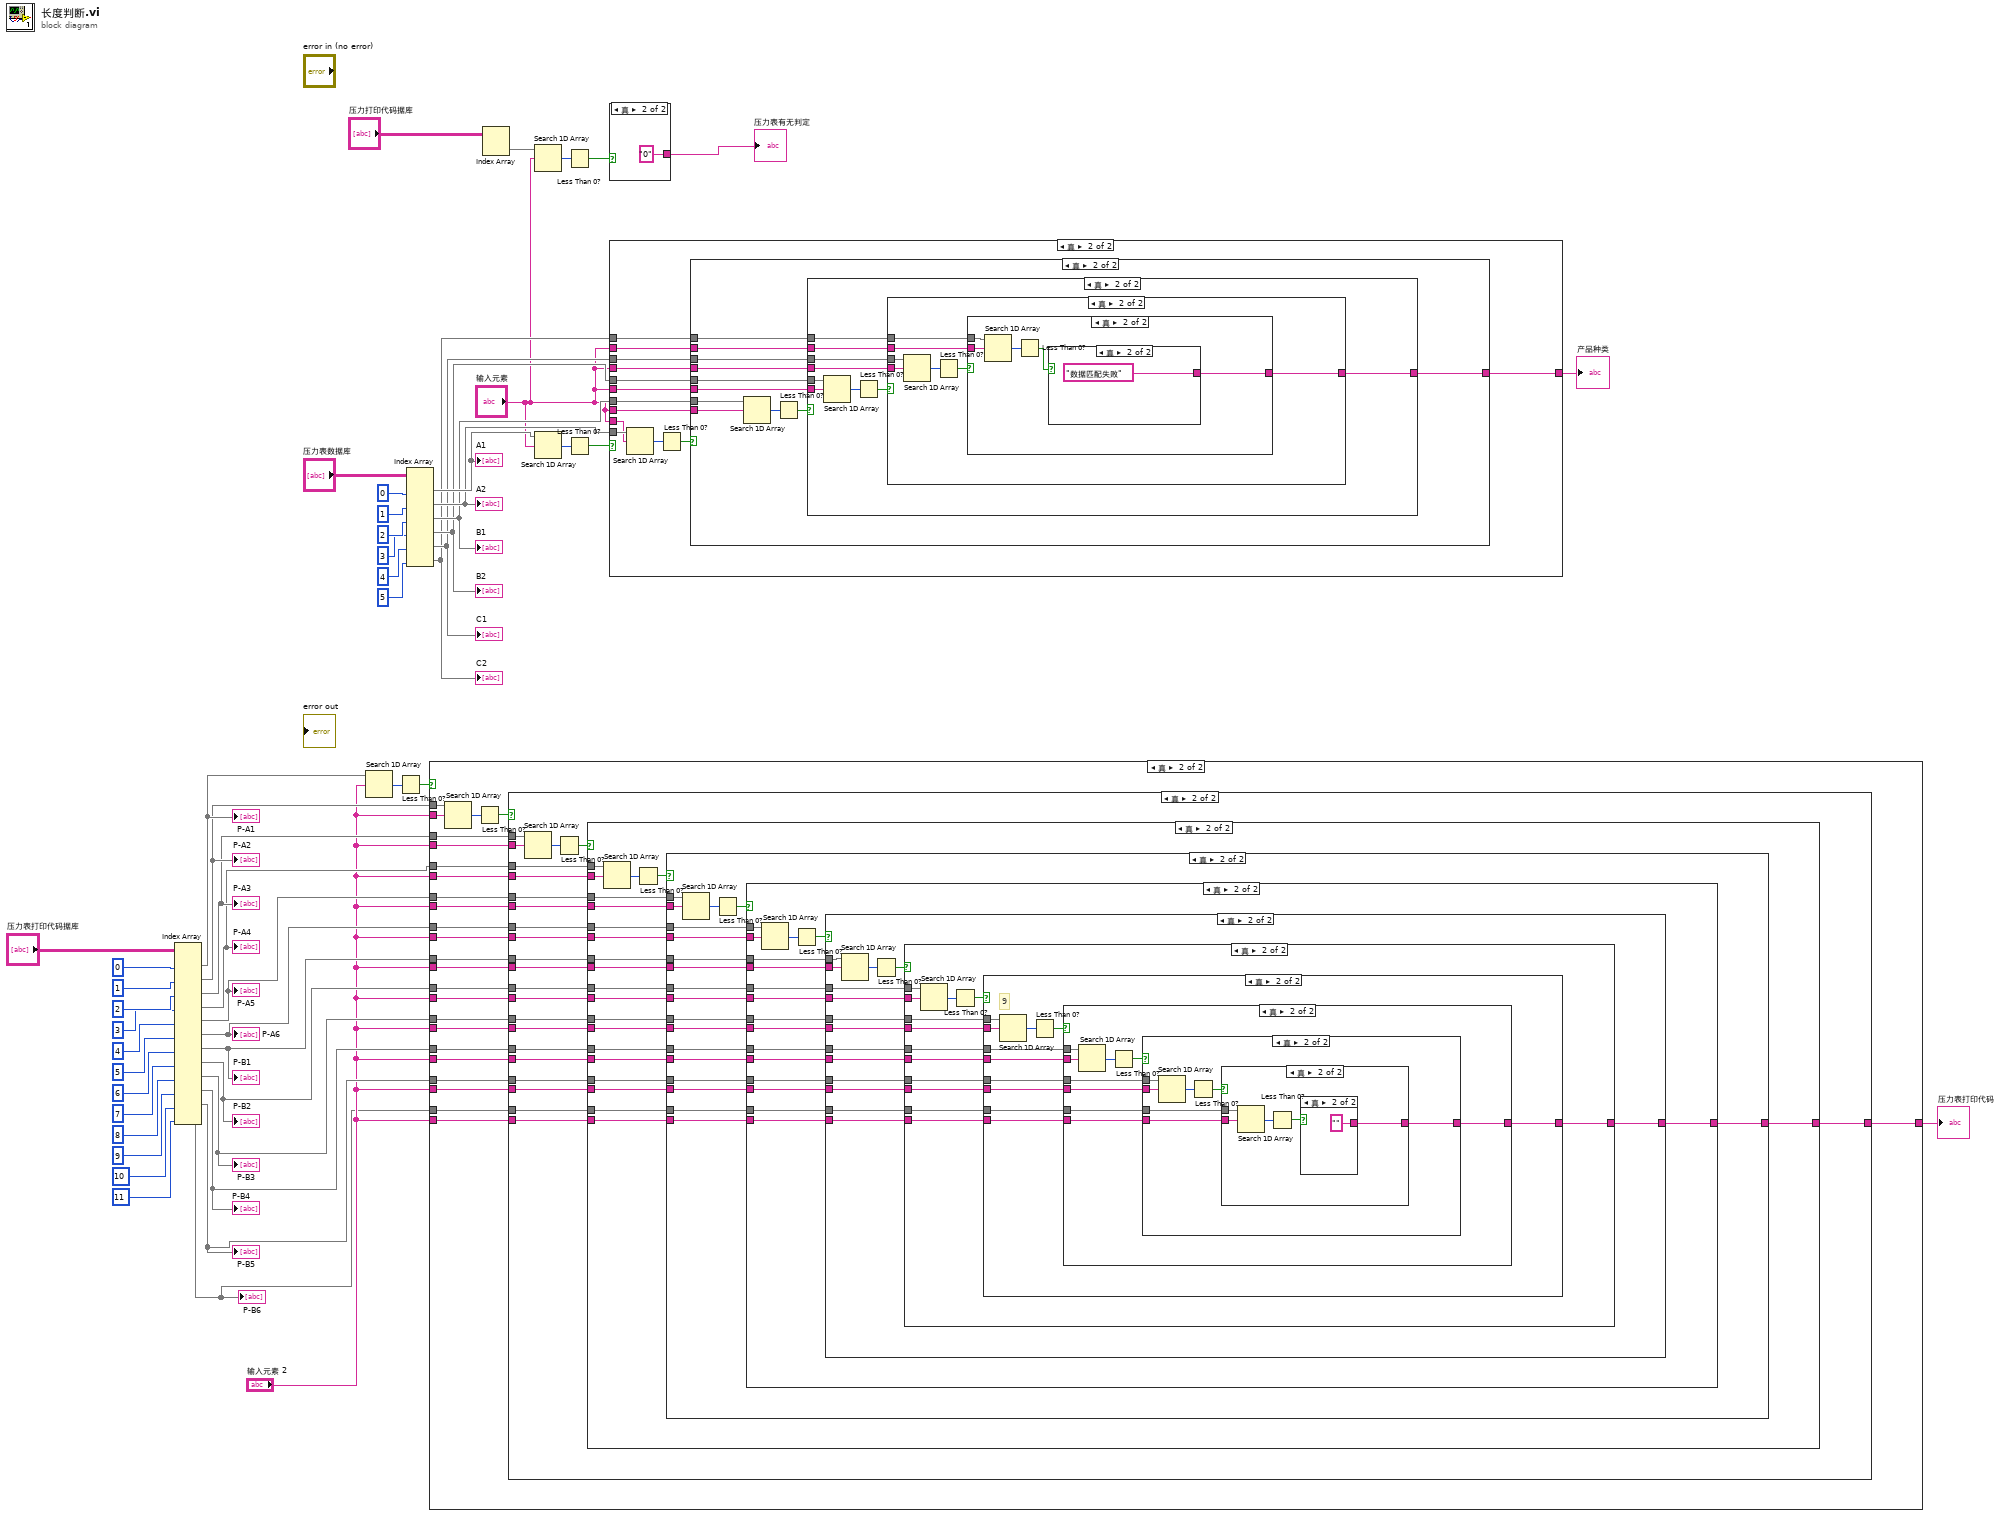
[diagram p0: block diagram]
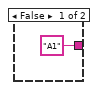
[diagram p2: hidden frame]
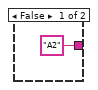
[diagram p3: hidden frame]
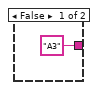
[diagram p4: hidden frame]
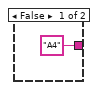
[diagram p5: hidden frame]
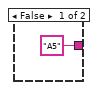
[diagram p6: hidden frame]
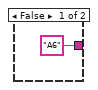
[diagram p7: hidden frame]
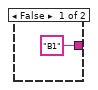
[diagram p8: hidden frame]
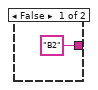
[diagram p9: hidden frame]
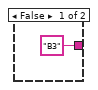
[diagram p10: hidden frame]
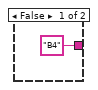
[diagram p11: hidden frame]
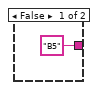
[diagram p12: hidden frame]
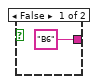
[diagram p13: hidden frame]
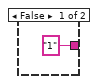
[diagram p14: hidden frame]
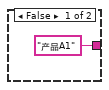
[diagram p15: hidden frame]
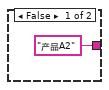
[diagram p16: hidden frame]
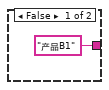
[diagram p17: hidden frame]
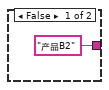
[diagram p18: hidden frame]
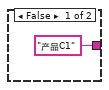
[diagram p19: hidden frame]
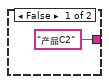
[diagram p20: hidden frame]
diagram:
  n1 = Index Array(array="压力表打印代码据库", index (col) #1=0 ("禁用的索引 (列)"), index (col) #2=1 ("索引 (列)"), index (col) #3=2 ("索引 (列)"), index (col) #4=3 ("索引 (列)"), index (col) #5=4 ("索引 (列)"), index (col) #6=5 ("索引 (列)"), index (col) #7=6 ("索引 (列)"), index (col) #8=7 ("索引 (列)"), index (col) #9=8 ("索引 (列)"), index (col) #10=9 ("索引 (列)"), index (col) #11=10 ("索引 (列)"), index (col) #12=11 ("索引 (列)")) -> (element #1=w13:string[], element #2=w12:string[], element #3=w11:string[], element #4=w10:string[], element #5=w9:string[], element #6=w8:string[], element #7=w7:string[], element #8=w6:string[], element #9=w5:string[], element #10=w4:string[], element #11=w3:string[], element #12=w1:string[])  [unwired: 12 in]
  "P-A1" <- w13
  "P-A2" <- w12
  "P-A3" <- w11
  "P-A4" <- w10
  "P-A5" <- w9
  "P-A6" <- w8
  "P-B1" <- w7
  "P-B2" <- w6
  "P-B3" <- w5
  "P-B4" <- w4
  "P-B5" <- w3
  "P-B6" <- w1
  n2 = Search 1D Array(1D array=w13, element="输入元素 2") -> (index of element=w18:i32)  [unwired: 1 in]
  n3 = Less Than 0?(x=w18) -> (x < 0?=w17:bool)
  n4 = Index Array(array="压力表数据库", index (col) #1=0 ("禁用的索引 (列)"), index (col) #2=1 ("索引 (列)"), index (col) #3=2 ("索引 (列)"), index (col) #4=3 ("索引 (列)"), index (col) #5=4 ("索引 (列)"), index (col) #6=5 ("索引 (列)")) -> (element #1=w47:string[], element #2=w44:string[], element #3=w43:string[], element #4=w33:string[], element #5=w32:string[], element #6=w31:string[])  [unwired: 6 in]
  "A1" <- w47
  "A2" <- w44
  "B1" <- w43
  "B2" <- w33
  "C1" <- w32
  "C2" <- w31
  n5 = case shown="真" w17 {
    tunnel: ["A1" w75] -> w14
    tunnel: "输入元素 2" -> [_ w74]
    tunnel: w12 -> [_ w73]
    tunnel: "输入元素 2" -> [_ w72]
    tunnel: w11 -> [_ w71]
    tunnel: "输入元素 2" -> [_ w70]
    tunnel: w10 -> [_ w69]
    tunnel: "输入元素 2" -> [_ w68]
    tunnel: w9 -> [_ w67]
    tunnel: "输入元素 2" -> [_ w66]
    tunnel: w8 -> [_ w65]
    tunnel: "输入元素 2" -> [_ w64]
    tunnel: w7 -> [_ w63]
    tunnel: "输入元素 2" -> [_ w62]
    tunnel: w6 -> [_ w61]
    tunnel: "输入元素 2" -> [_ w60]
    tunnel: w5 -> [_ w59]
    tunnel: "输入元素 2" -> [_ w58]
    tunnel: w4 -> [_ w57]
    tunnel: "输入元素 2" -> [_ w56]
    tunnel: w3 -> [_ w55]
    tunnel: "输入元素 2" -> [_ w54]
    tunnel: w1 -> [_ w53]
    frame False {
    }
    frame True {
      n6 = Search 1D Array(1D array=w73, element=w74) -> (index of element=w77:i32)  [unwired: 1 in]
      n7 = Less Than 0?(x=w77) -> (x < 0?=w76:bool)
      n8 = case shown="真" w76 {
        tunnel: ["A2" w99] -> w75
        tunnel: w72 -> [_ w98]
        tunnel: w71 -> [_ w97]
        tunnel: w70 -> [_ w96]
        tunnel: w69 -> [_ w95]
        tunnel: w68 -> [_ w94]
        tunnel: w67 -> [_ w93]
        tunnel: w66 -> [_ w92]
        tunnel: w65 -> [_ w91]
        tunnel: w64 -> [_ w90]
        tunnel: w63 -> [_ w89]
        tunnel: w62 -> [_ w88]
        tunnel: w61 -> [_ w87]
        tunnel: w60 -> [_ w86]
        tunnel: w59 -> [_ w85]
        tunnel: w58 -> [_ w84]
        tunnel: w57 -> [_ w83]
        tunnel: w56 -> [_ w82]
        tunnel: w55 -> [_ w81]
        tunnel: w54 -> [_ w80]
        tunnel: w53 -> [_ w79]
        frame False {
        }
        frame True {
          n9 = Search 1D Array(1D array=w97, element=w98) -> (index of element=w101:i32)  [unwired: 1 in]
          n10 = Less Than 0?(x=w101) -> (x < 0?=w100:bool)
          n11 = case shown="真" w100 {
            tunnel: ["A3" w121] -> w99
            tunnel: w96 -> [_ w120]
            tunnel: w95 -> [_ w119]
            tunnel: w94 -> [_ w118]
            tunnel: w93 -> [_ w117]
            tunnel: w92 -> [_ w116]
            tunnel: w91 -> [_ w115]
            tunnel: w90 -> [_ w114]
            tunnel: w89 -> [_ w113]
            tunnel: w88 -> [_ w112]
            tunnel: w87 -> [_ w111]
            tunnel: w86 -> [_ w110]
            tunnel: w85 -> [_ w109]
            tunnel: w84 -> [_ w108]
            tunnel: w83 -> [_ w107]
            tunnel: w82 -> [_ w106]
            tunnel: w81 -> [_ w105]
            tunnel: w80 -> [_ w104]
            tunnel: w79 -> [_ w103]
            frame False {
            }
            frame True {
              n12 = Search 1D Array(1D array=w119, element=w120) -> (index of element=w123:i32)  [unwired: 1 in]
              n13 = Less Than 0?(x=w123) -> (x < 0?=w122:bool)
              n14 = case shown="真" w122 {
                tunnel: ["A4" w143] -> w121
                tunnel: w118 -> [_ w140]
                tunnel: w117 -> [_ w139]
                tunnel: w116 -> [_ w138]
                tunnel: w115 -> [_ w137]
                tunnel: w114 -> [_ w136]
                tunnel: w113 -> [_ w135]
                tunnel: w112 -> [_ w134]
                tunnel: w111 -> [_ w133]
                tunnel: w110 -> [_ w132]
                tunnel: w109 -> [_ w131]
                tunnel: w108 -> [_ w130]
                tunnel: w107 -> [_ w129]
                tunnel: w106 -> [_ w128]
                tunnel: w105 -> [_ w127]
                tunnel: w104 -> [_ w126]
                tunnel: w103 -> [_ w125]
                frame False {
                }
                frame True {
                  n15 = Search 1D Array(1D array=w139, element=w140) -> (index of element=w142:i32)  [unwired: 1 in]
                  n16 = Less Than 0?(x=w142) -> (x < 0?=w141:bool)
                  n17 = case shown="真" w141 {
                    tunnel: ["A5" w161] -> w143
                    tunnel: w138 -> [_ w158]
                    tunnel: w137 -> [_ w157]
                    tunnel: w136 -> [_ w156]
                    tunnel: w135 -> [_ w155]
                    tunnel: w134 -> [_ w154]
                    tunnel: w133 -> [_ w153]
                    tunnel: w132 -> [_ w152]
                    tunnel: w131 -> [_ w151]
                    tunnel: w130 -> [_ w150]
                    tunnel: w129 -> [_ w149]
                    tunnel: w128 -> [_ w148]
                    tunnel: w127 -> [_ w147]
                    tunnel: w126 -> [_ w146]
                    tunnel: w125 -> [_ w145]
                    frame False {
                    }
                    frame True {
                      n18 = Search 1D Array(1D array=w157, element=w158) -> (index of element=w160:i32)  [unwired: 1 in]
                      n19 = Less Than 0?(x=w160) -> (x < 0?=w159:bool)
                      n20 = case shown="真" w159 {
                        tunnel: ["A6" w177] -> w161
                        tunnel: w156 -> [_ w174]
                        tunnel: w155 -> [_ w173]
                        tunnel: w154 -> [_ w172]
                        tunnel: w153 -> [_ w171]
                        tunnel: w152 -> [_ w170]
                        tunnel: w151 -> [_ w169]
                        tunnel: w150 -> [_ w168]
                        tunnel: w149 -> [_ w167]
                        tunnel: w148 -> [_ w166]
                        tunnel: w147 -> [_ w165]
                        tunnel: w146 -> [_ w164]
                        tunnel: w145 -> [_ w163]
                        frame False {
                        }
                        frame True {
                          n21 = Search 1D Array(1D array=w173, element=w174) -> (index of element=w176:i32)  [unwired: 1 in]
                          n22 = Less Than 0?(x=w176) -> (x < 0?=w175:bool)
                          n23 = case shown="真" w175 {
                            tunnel: ["B1" w191] -> w177
                            tunnel: w172 -> [_ w188]
                            tunnel: w171 -> [_ w187]
                            tunnel: w170 -> [_ w186]
                            tunnel: w169 -> [_ w185]
                            tunnel: w168 -> [_ w184]
                            tunnel: w167 -> [_ w183]
                            tunnel: w166 -> [_ w182]
                            tunnel: w165 -> [_ w181]
                            tunnel: w164 -> [_ w180]
                            tunnel: w163 -> [_ w179]
                            frame False {
                            }
                            frame True {
                              n24 = Search 1D Array(1D array=w187, element=w188) -> (index of element=w190:i32)  [unwired: 1 in]
                              n25 = Less Than 0?(x=w190) -> (x < 0?=w189:bool)
                              n26 = case shown="真" w189 {
                                tunnel: ["B2" w203] -> w191
                                tunnel: w186 -> [_ w200]
                                tunnel: w185 -> [_ w199]
                                tunnel: w184 -> [_ w198]
                                tunnel: w183 -> [_ w197]
                                tunnel: w182 -> [_ w196]
                                tunnel: w181 -> [_ w195]
                                tunnel: w180 -> [_ w194]
                                tunnel: w179 -> [_ w193]
                                frame False {
                                }
                                frame True {
                                # "9"
                                n27 = Search 1D Array(1D array=w199, element=w200) -> (index of element=w202:i32)  [unwired: 1 in]
                                n28 = Less Than 0?(x=w202) -> (x < 0?=w201:bool)
                                n29 = case shown="真" w201 {
                                tunnel: ["B3" w213] -> w203
                                tunnel: w198 -> [_ w210]
                                tunnel: w197 -> [_ w209]
                                tunnel: w196 -> [_ w208]
                                tunnel: w195 -> [_ w207]
                                tunnel: w194 -> [_ w206]
                                tunnel: w193 -> [_ w205]
                                frame False {
                                }
                                frame True {
                                n30 = Search 1D Array(1D array=w209, element=w210) -> (index of element=w212:i32)  [unwired: 1 in]
                                n31 = Less Than 0?(x=w212) -> (x < 0?=w211:bool)
                                n32 = case shown="真" w211 {
                                tunnel: ["B4" w221] -> w213
                                tunnel: w208 -> [_ w218]
                                tunnel: w207 -> [_ w217]
                                tunnel: w206 -> [_ w216]
                                tunnel: w205 -> [_ w215]
                                frame False {
                                }
                                frame True {
                                n33 = Search 1D Array(1D array=w217, element=w218) -> (index of element=w220:i32)  [unwired: 1 in]
                                n34 = Less Than 0?(x=w220) -> (x < 0?=w219:bool)
                                n35 = case shown="真" w219 {
                                tunnel: ["B5" w227] -> w221
                                tunnel: w216 -> [_ w224]
                                tunnel: w215 -> [_ w223]
                                frame False {
                                }
                                frame True {
                                n36 = Search 1D Array(1D array=w223, element=w224) -> (index of element=w226:i32)  [unwired: 1 in]
                                n37 = Less Than 0?(x=w226) -> (x < 0?=w225:bool)
                                n38 = case shown="真" w225 {
                                tunnel: ["B6" ""] -> w227
                                frame False {
                                }
                                frame True {
                                }
                                }
                                }
                                }
                                }
                                }
                                }
                                }
                                }
                              }
                            }
                          }
                        }
                      }
                    }
                  }
                }
              }
            }
          }
        }
      }
    }
  }
  "压力表打印代码" <- w14
  n39 = Index Array(array="压力打印代码据库") -> (element=w40:string[])  [unwired: 2 in]
  n40 = Search 1D Array(1D array=w40, element="输入元素") -> (index of element=w42:i32)  [unwired: 1 in]
  n41 = Search 1D Array(1D array=w47, element="输入元素") -> (index of element=w46:i32)  [unwired: 1 in]
  n42 = Less Than 0?(x=w42) -> (x < 0?=w39:bool)
  n43 = Less Than 0?(x=w46) -> (x < 0?=w45:bool)
  n44 = case shown="真" w39 {
    tunnel: ["1" "0"] -> w38
    frame False {
    }
    frame True {
    }
  }
  "压力表有无判定" <- w38
  n45 = case shown="真" w45 {
    tunnel: w44 -> [_ w244]
    tunnel: "输入元素" -> [_ w243]
    tunnel: w43 -> [_ w241]
    tunnel: "输入元素" -> [_ w240]
    tunnel: ["产品A1" w239] -> w37
    tunnel: w33 -> [_ w238]
    tunnel: w32 -> [_ w237]
    tunnel: w31 -> [_ w236]
    tunnel: "输入元素" -> [_ w235]
    tunnel: "输入元素" -> [_ w234]
    tunnel: "输入元素" -> [_ w233]
    frame False {
    }
    frame True {
      n46 = Search 1D Array(1D array=w244, element=w243) -> (index of element=w245:i32)  [unwired: 1 in]
      n47 = Less Than 0?(x=w245) -> (x < 0?=w242:bool)
      n48 = case shown="真" w242 {
        tunnel: w241 -> [_ w256]
        tunnel: w240 -> [_ w255]
        tunnel: ["产品A2" w253] -> w239
        tunnel: w238 -> [_ w252]
        tunnel: w237 -> [_ w251]
        tunnel: w236 -> [_ w250]
        tunnel: w235 -> [_ w249]
        tunnel: w234 -> [_ w248]
        tunnel: w233 -> [_ w247]
        frame False {
        }
        frame True {
          n49 = Search 1D Array(1D array=w256, element=w255) -> (index of element=w257:i32)  [unwired: 1 in]
          n50 = Less Than 0?(x=w257) -> (x < 0?=w254:bool)
          n51 = case shown="真" w254 {
            tunnel: ["产品B1" w264] -> w253
            tunnel: w252 -> [_ w266]
            tunnel: w251 -> [_ w263]
            tunnel: w250 -> [_ w262]
            tunnel: w249 -> [_ w261]
            tunnel: w248 -> [_ w260]
            tunnel: w247 -> [_ w259]
            frame False {
            }
            frame True {
              n52 = Search 1D Array(1D array=w266, element=w261) -> (index of element=w267:i32)  [unwired: 1 in]
              n53 = Less Than 0?(x=w267) -> (x < 0?=w265:bool)
              n54 = case shown="真" w265 {
                tunnel: ["产品B2" w274] -> w264
                tunnel: w263 -> [_ w272]
                tunnel: w262 -> [_ w271]
                tunnel: w260 -> [_ w270]
                tunnel: w259 -> [_ w269]
                frame False {
                }
                frame True {
                  n55 = Search 1D Array(1D array=w272, element=w270) -> (index of element=w275:i32)  [unwired: 1 in]
                  n56 = Less Than 0?(x=w275) -> (x < 0?=w273:bool)
                  n57 = case shown="真" w273 {
                    tunnel: ["产品C1" w278] -> w274
                    tunnel: w271 -> [_ w280]
                    tunnel: w269 -> [_ w277]
                    frame False {
                    }
                    frame True {
                      n58 = Search 1D Array(1D array=w280, element=w277) -> (index of element=w281:i32)  [unwired: 1 in]
                      n59 = Less Than 0?(x=w281) -> (x < 0?=w279:bool)
                      n60 = case shown="真" w279 {
                        tunnel: ["产品C2" "数据匹配失败"] -> w278
                        frame False {
                        }
                        frame True {
                        }
                      }
                    }
                  }
                }
              }
            }
          }
        }
      }
    }
  }
  "产品种类" <- w37
